vi "Helper SubVI - Vector Interpolation.vi"(6 "phase 0":dbl[](array[numeric]), 7 "hop":i32=256, 8 "N":i32=1024, 9 "new time instance (t)":dbl, 10 "FFT (t1)":cdb[](array[numeric]), 11 "FFT (t0)":cdb[](array[numeric])) -> (3 "interpolation":cdb[](array[numeric]))   [LabVIEW 2023]
doc: "Performs vector interpolation."
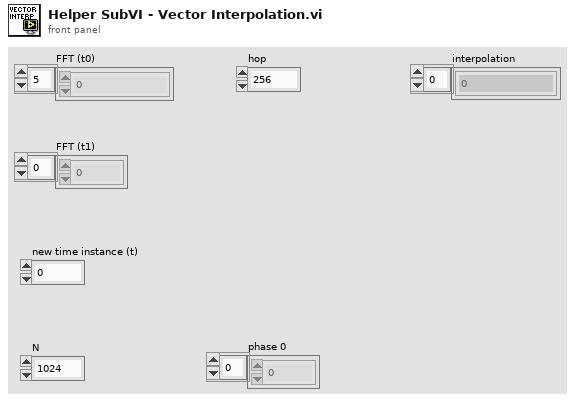
[diagram p1: front panel]
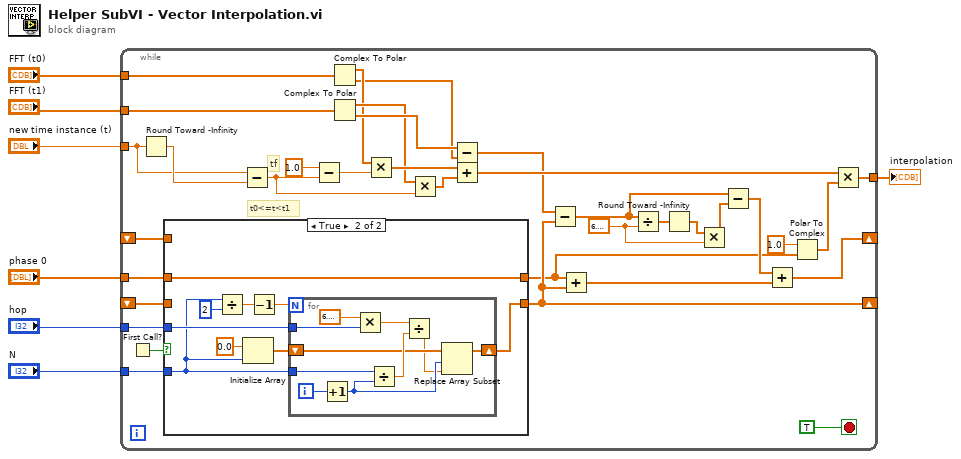
[diagram p0: block diagram]
diagram:
  n1 = while {
    shift-right: [w11] -> _
    shift-left: _ -> [w18]
    shift-right: [w19] -> _
    shift-left: _ -> [w20]
    tunnel: "hop" -> [w17]
    tunnel: "FFT (t0)" -> [w16]
    tunnel: "FFT (t1)" -> [w15]
    tunnel: "new time instance (t)" -> [w14]
    tunnel: [w13] -> w3
    tunnel: "phase 0" -> [w10]
    tunnel: "N" -> [w9]
    stop <- TRUE stop-if-true
    w35 = 6.283185307179586 ("Pi Multiplied By 2")
    # "t0<=t<t1"
    # "tf"
    n2 = First Call?() -> (First Call?: T/F=w21:bool)
    n3 = Round Toward -Infinity(1:w14) -> (0:w23:dbl)
    n4 = case shown="True" w21 {
      tunnel: [w44 w49] -> w19
      tunnel: w20 -> [w44 _]
      tunnel: [w43 w46] -> w8
      tunnel: w18 -> [w43 _]
      tunnel: w17 -> [_ w48]
      tunnel: w10 -> [_ w46]
      tunnel: w9 -> [_ w45]
      frame False {
      }
      frame True {
        n5 = Divide(x=w45, y=2) -> (x/y=w47:dbl)
        n6 = Initialize Array(0.0 ("element"), w45) -> (w50:dbl[])
        n7 = Decrement(x=w47) -> (x-1=w52:dbl)
        n8 = for {
          N: w52 -> [_]
          shift-right: [w54] -> w49
          shift-left: w50 -> [w57]
          tunnel: w48 -> [w62]
          tunnel: w45 -> [w61]
          i -> [w60]
          n9 = Increment(x=w60) -> (x+1=w56:i32)
          n10 = Multiply(x=6.283185307179586 ("Pi Multiplied By 2"), y=w62) -> (x*y=w59:dbl)
          n11 = Divide(x=w61, y=w56) -> (x/y=w58:dbl)
          n12 = Divide(x=w59, y=w58) -> (x/y=w55:dbl)
          n13 = Replace Array Subset(array=w57, new element=w55, index=w56) -> (w54:dbl[])
        }
      }
    }
    n14 = Subtract(x=w14, y=w23) -> (x-y=w28:dbl)
    n15 = Subtract(x=1.0, y=w28) -> (x-y=w25:dbl)
    n16 = Complex To Polar(r * e^(i*theta)=w16) -> (r=w26:dbl[], theta=w12:dbl[])
    n17 = Complex To Polar(r * e^(i*theta)=w15) -> (r=w27:dbl[], theta=w42:dbl[])
    n18 = Multiply(x=w26, y=w25) -> (x*y=w29:dbl[])
    n19 = Multiply(x=w27, y=w28) -> (x*y=w30:dbl[])
    n20 = Subtract(x=w42, y=w12) -> (x-y=w31:dbl[])
    n21 = Add(x=w29, y=w30) -> (x+y=w38:dbl[])
    n22 = Subtract(x=w31, y=w19) -> (x-y=w33:dbl[])
    n23 = Add(x=w8, y=w19) -> (x+y=w40:dbl[])
    n24 = Divide(x=w33, y=w35) -> (x/y=w32:dbl[])
    n25 = Round Toward -Infinity(1:w32) -> (0:w34:dbl[])
    n26 = Multiply(x=w34, y=w35) -> (x*y=w36:dbl[])
    n27 = Subtract(x=w33, y=w36) -> (x-y=w41:dbl[])
    n28 = Add(x=w41, y=w40) -> (x+y=w11:dbl[])
    n29 = Polar To Complex(1:w8, 2:1.0 ("r")) -> (0:w39:cdb[])
    n30 = Multiply(x=w38, y=w39) -> (x*y=w13:cdb[])
  }
  "interpolation" <- w3
